vi "SP Complex Inverse Matrix (LU).vi"(3 "A":T1) -> (0 "error":i32, 1 "Inverse Matrix":T1)   [LabVIEW 2011]
doc: "Finds the <B>Inverse Matrix</B>, if it exists, of the <B>Input Matrix</B>, using LU factorization."
uses:
  TypeDefs/SP Complex Matrix.ctl
  Program Files/National Instruments/LabVIEW 2011/resource/lvanlys.dll
panel:
  # "Complex Inverse Matrix (LU)"
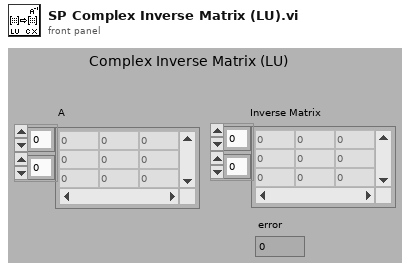
[diagram p1: front panel]
types:
  T1 = typedef "SP Complex Matrix.ctl" = cdb[][]
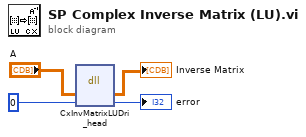
[diagram p0: block diagram]
diagram:
  n1 = dll-call lib="C:/Program Files/National Instruments/LabVIEW 2011/resource/lvanlys.*" fn="CxInvMatrixLUDri_head"("A"="A", 0) -> ("A"=→"Inverse Matrix":T1, →"error":i32)  [unwired: 3 in, 3 out]
